vi "Parse Installed Files.vi"(7 "Package Name":string, 8 "Error In":errorcluster, 10 "Files Installed":path[](array[path]), 11 "Dependecy Config in":T1) -> (0 "Error Out":errorcluster, 2 "Config Found?":bool, 3 "Dependecy Config out":T1)   [LabVIEW 2011, in "LMH-Toolbox.lvlib" / "LMH-Installer Tools.lvlib"]
uses:
  LMH-Installer Tools.lvlib
  Type Defs/Dependency Config.ctl
  Type Defs/Dependecy.ctl
  Web/Type Defs/Download Task.ctl
  Web/LMH-Web.lvlib
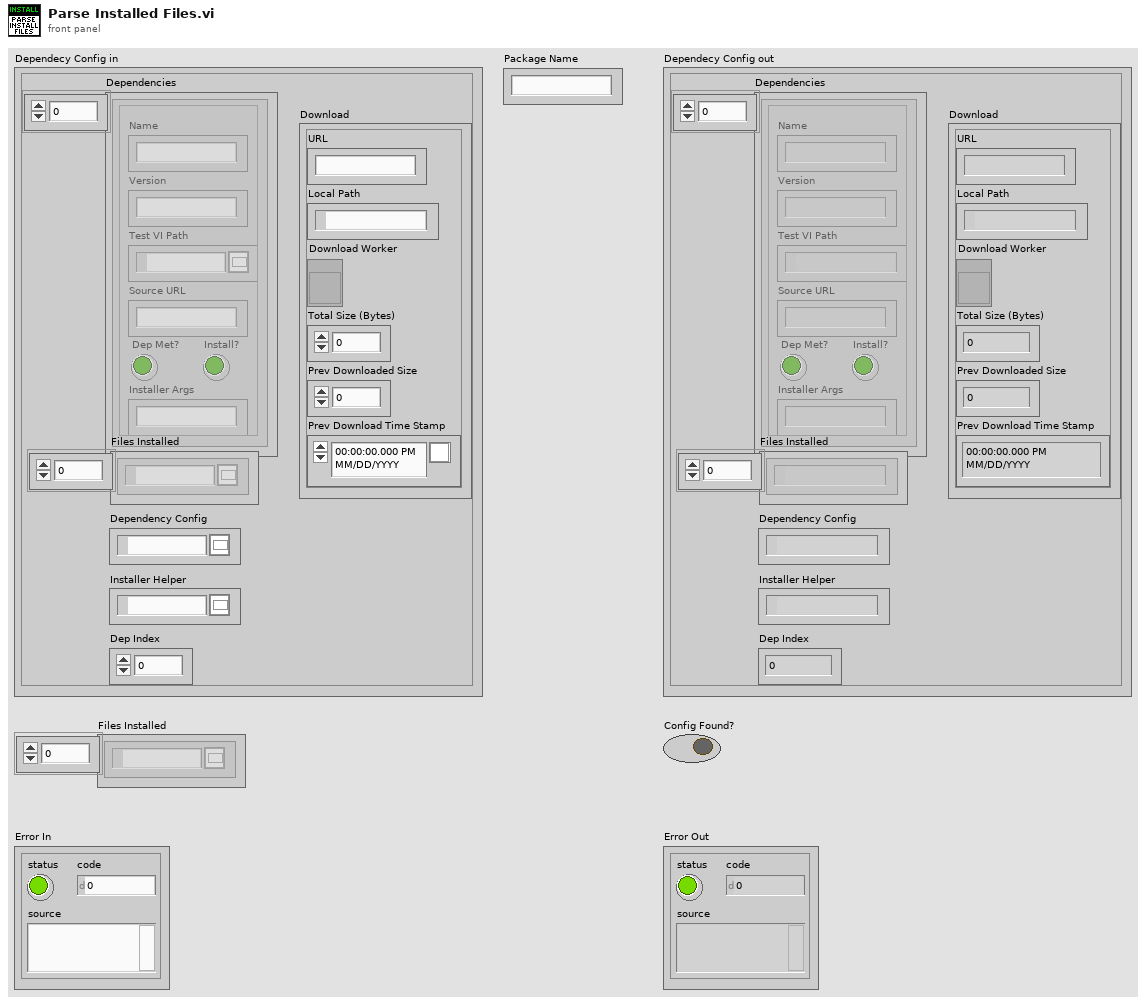
[diagram p1: front panel]
types:
  T1 = typedef "LMH-Toolbox.lvlib/LMH-Installer Tools.lvlib/Dependency Config.ctl" = cluster{"Dependencies":T2[], "Files Installed":path[], "Dependency Config":path, "Installer Helper":path, "Dep Index":i32, "Download":T3}
  T2 = typedef "LMH-Toolbox.lvlib/LMH-Installer Tools.lvlib/Dependecy.ctl" = cluster{"Name":string, "Version":string, "Test VI Path":path, "Source URL":string, "Dep Met?":bool, "Install?":bool, "Installer Args":string}
  T3 = typedef "LMH-Toolbox.lvlib/LMH-Web.lvlib/Download Task.ctl" = cluster{"URL":string, "Local Path":path, "Download Worker":refnum<vi>, "Total Size (Bytes)":u64, "Prev Downloaded Size":u64, "Prev Download Time Stamp":timestamp}
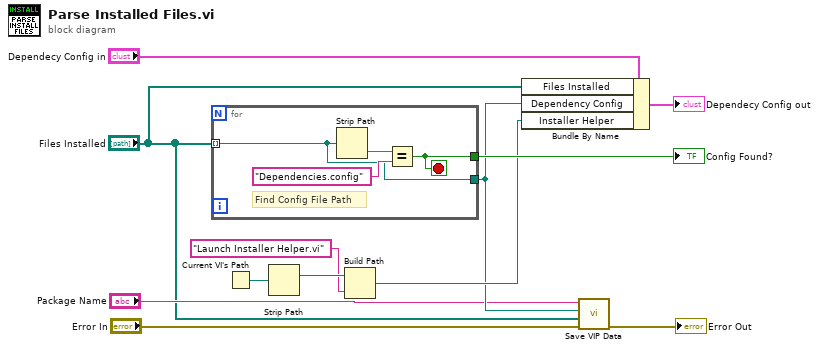
[diagram p0: block diagram]
diagram:
  n1 = for {
    tunnel: "Files Installed" -> [w13] mode=indexing
    tunnel: [w14] -> w10
    tunnel: [w13] -> w5
    stop <- w14 stop-if-true
    # "Find Config File Path"
    n2 = Strip Path(path=w13) -> (name=w16:string)  [unwired: 1 out]
    n3 = Equal?(x=w16, y="Dependencies.config") -> (x = y?=w14:bool)
  }
  "Config Found?" <- w10
  n4 = Current VI's Path() -> (path=w8:path)
  n5 = Strip Path(path=w8) -> (stripped path=w9:path)  [unwired: 1 out]
  n6 = Build Path(base path=w9, name or relative path="Launch Installer Helper.vi") -> (appended path=w7:path)
  n7 = Bundle By Name(cluster="Dependecy Config in", "Files Installed"="Files Installed", "Dependency Config"=w5, "Installer Helper"=w7) -> (→"Dependecy Config out":T1)
  n8 = call "Save VIP Data.vi"("Error In"="Error In", "Files Installed"="Files Installed", "Dependencies.config"=w5, "Package Name"="Package Name") -> ("Error Out"=→"Error Out":errorcluster)  [unwired: 7 in]
